vi "Read Payload Mask.vi"(8 "error in":errorcluster, 11 "OOB in":refnum<class "CIFOutOfBand.lvclass">) -> (0 "error out":errorcluster, 2 "Cases to Skip Payload":u8[](array[numeric]), 3 "OOB out":refnum<class "CIFOutOfBand.lvclass">)   [LabVIEW 2021, in "CIFOutOfBand.lvclass"]
uses:
  CIFOutOfBand.lvclass
  CIFOutOfBand.lvclass/CIFOutOfBand.ctl
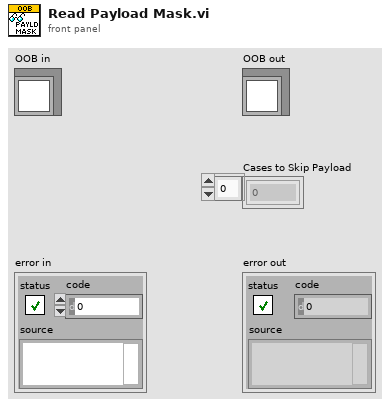
[diagram p1: front panel]
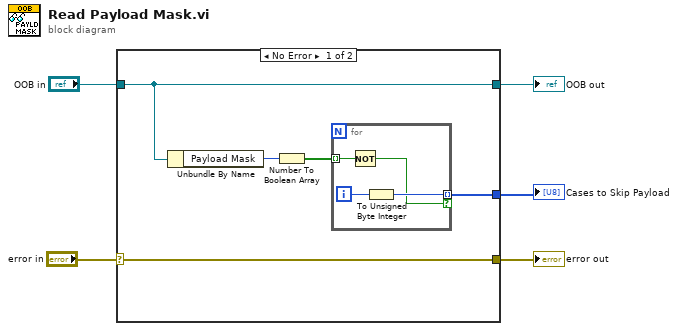
[diagram p0: block diagram]
diagram:
  n1 = case shown="No Error" "error in" {
    selector: "error in" -> [w10 w15]
    tunnel: [w10 w15] -> w4
    tunnel: [w9 w16] -> w2
    tunnel: "OOB in" -> [w9 w16]
    tunnel: [w6 _] -> w1
    frame No Error {
      n2 = Unbundle By Name(w9) -> ("Payload Mask"=w8:u64)
      n3 = Number To Boolean Array(number=w8) -> (Boolean array=w7:bool[])
      n4 = for {
        tunnel: w7 -> [w12] mode=indexing
        tunnel: [w13] -> w6 mode=indexing if=w11
        i -> [w14]
        n5 = Not(x=w12) -> (.not. x?=w11:bool)
        n6 = To Unsigned Byte Integer(number=w14) -> (unsigned 8bit integer=w13:u8)
      }
    }
    frame Error {
    }
  }
  "error out" <- w4
  "OOB out" <- w2
  "Cases to Skip Payload" <- w1
